vi "Set_K2400_Range.vi"(8 "error in (no error)":errorcluster, 10 "Desired Voltage":dbl format="%_6g") -> (0 "error out":errorcluster)   [LabVIEW 2020]
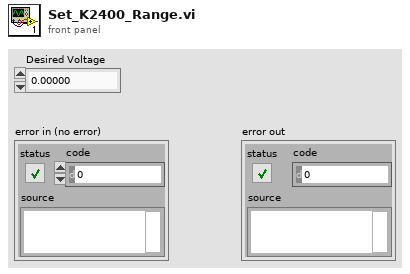
[diagram p1: front panel]
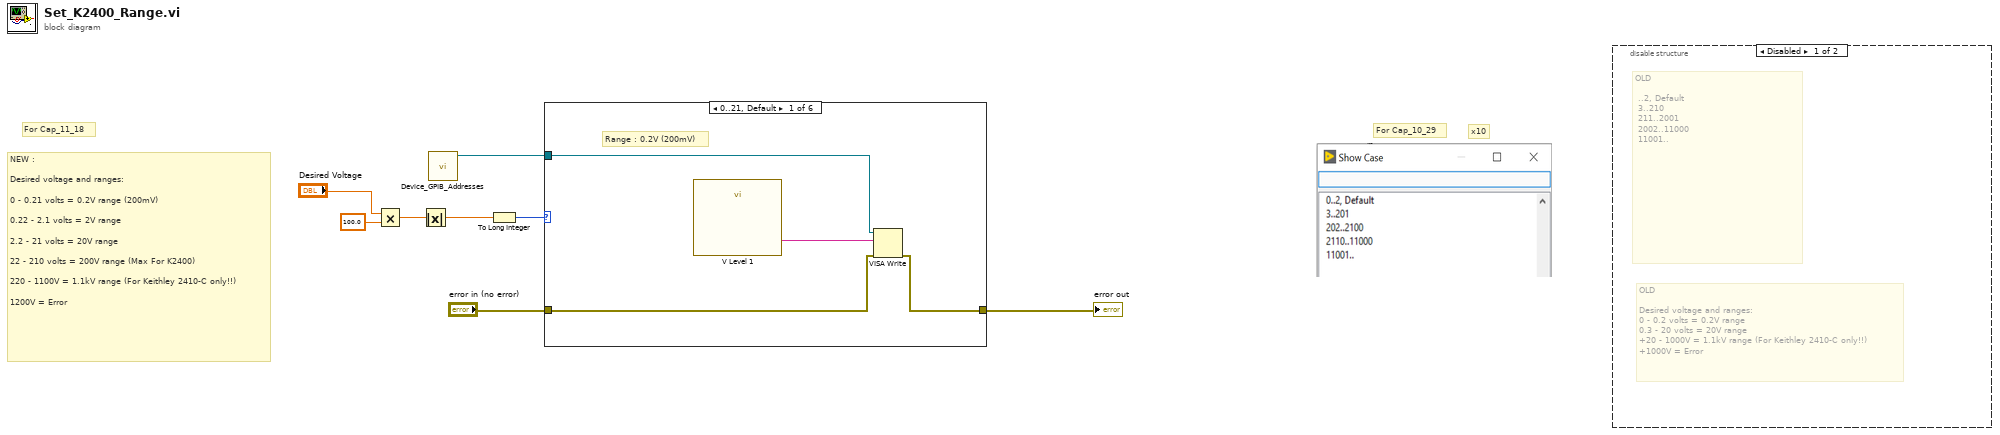
[diagram p0: block diagram]
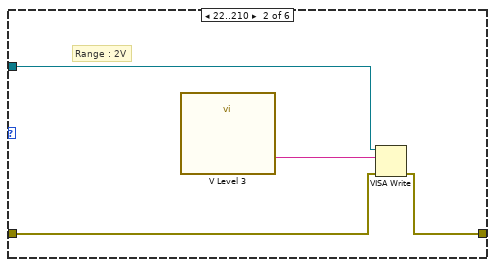
[diagram p3: hidden frame]
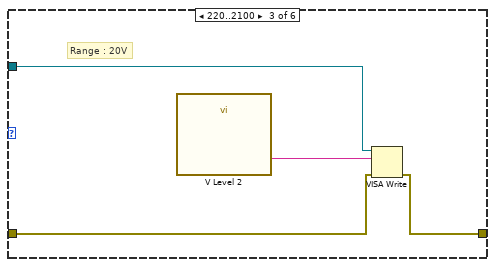
[diagram p4: hidden frame]
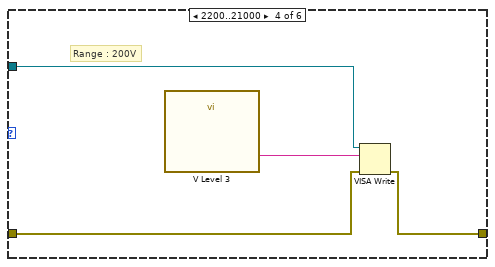
[diagram p5: hidden frame]
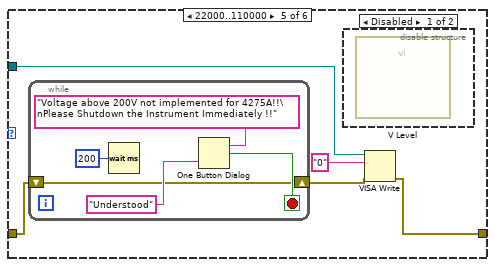
[diagram p6: hidden frame]
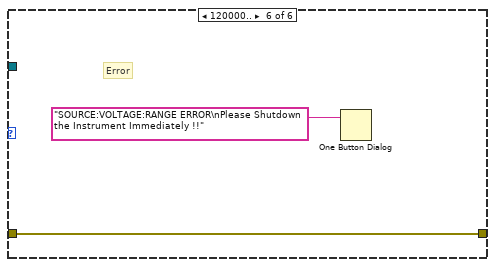
[diagram p8: hidden frame]
diagram:
  # "x10"
  # "For Cap_11_18"
  # "For Cap_10_29"
  # "NEW :\n\nDesired voltage and ranges:\n\n0 - 0.21 volts = 0.2V range (200mV)\n\n0.22 - 2.1 volts = 2V range\n\n2.2 - 21 volts = 20V range\n\n22 - 210 volts = 200V range (Max For K2400)\n\n220 - 1100V = 1.1kV range (For Keithley 2410-C only!!)\n \n1200V = Error"
  n1 = Multiply(x="Desired Voltage", y=100.0) -> (x*y=w3:dbl)
  n2 = Absolute Value(x=w3) -> (abs(x)=w2:dbl)
  n3 = call "Device_GPIB_Addresses.vi"() -> ("Keithley 2400 Address"=w4:refnum<visa-resource-name>)  [unwired: 9 in, 2 out]
  n4 = To Long Integer(number=w2) -> (32bit integer=w6:i32)
  n5 = case shown="0..21, Default" w6 {
    tunnel: w4 -> [w11 w15 w19 w23 w29 _]
    tunnel: "error in (no error)" -> [w10 w14 w18 w22 w25 w36]
    tunnel: [w9 w13 w17 w21 w28 w36] -> w1
    frame 0..21, Default {
      # "Range : 0.2V (200mV)"
      n6 = call "V Level 1"() -> ("Result"=w12:string)  [unwired: 4 in, 11 out]
      n7 = VISA Write(VISA resource name=w11, write buffer=w12, error in (no error)=w10) -> (error out=w9:errorcluster)  [unwired: 2 out]
    }
    frame 22..210 {
      # "Range : 2V"
      n8 = call "V Level 3"() -> ("Result"=w16:string)  [unwired: 4 in, 11 out]
      n9 = VISA Write(VISA resource name=w15, write buffer=w16, error in (no error)=w14) -> (error out=w13:errorcluster)  [unwired: 2 out]
    }
    frame 220..2100 {
      # "Range : 20V"
      n10 = call "V Level 2"() -> ("Result"=w20:string)  [unwired: 4 in, 11 out]
      n11 = VISA Write(VISA resource name=w19, write buffer=w20, error in (no error)=w18) -> (error out=w17:errorcluster)  [unwired: 2 out]
    }
    frame 2200..21000 {
      # "Range : 200V"
      n12 = call "V Level 3"() -> ("Result"=w24:string)  [unwired: 4 in, 11 out]
      n13 = VISA Write(VISA resource name=w23, write buffer=w24, error in (no error)=w22) -> (error out=w21:errorcluster)  [unwired: 2 out]
    }
    frame 22000..110000 {
      n14 = while {
        shift-right: [w30] -> w26
        shift-left: w25 -> [w30]
        stop <- w33 stop-if-true
        n15 = Wait (ms)(milliseconds to wait=u32 200) -> ()  [unwired: 1 out]
        n16 = One Button Dialog(message="Voltage above 200V not implemented for 4275A!!\nPlease Shutdown the Instrument Immediately !!", button name ("OK")="Understood") -> (true=w33:bool)
      }
      n17 = disable-structure shown="Disabled" {
        frame Disabled {
          n18 = call "V Level"() -> ()  [unwired: 4 in, 12 out]
        }
        frame Enabled {
        }
      }
      n19 = VISA Write(VISA resource name=w29, write buffer="0", error in (no error)=w26) -> (error out=w28:errorcluster)  [unwired: 2 out]
    }
    frame 120000.. {
      # "Error"
      n20 = One Button Dialog(message="SOURCE:VOLTAGE:RANGE ERROR\nPlease Shutdown the Instrument Immediately !!") -> ()  [unwired: 1 in, 1 out]
    }
  }
  "error out" <- w1
  n21 = disable-structure shown="Disabled" {
    frame Disabled {
      # "OLD\n\n ..2, Default\n 3..210 \n 211..2001 \n 2002..11000\n 11001.."
      # "OLD\n\nDesired voltage and ranges:\n0 - 0.2 volts = 0.2V range\n0.3 - 20 volts = 20V range\n+20 - 1000V = 1.1kV range (For Keithley 2410-C only!!) \n+1000V = Error"
    }
    frame Enabled {
    }
  }
